vi "Count Change.vi"(1 "reset":bool, 2 "X":variant, 3 "Y":variant) -> (0 "Out":dbl)   [LabVIEW 2019]
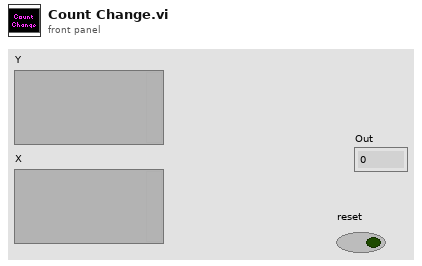
[diagram p1: front panel]
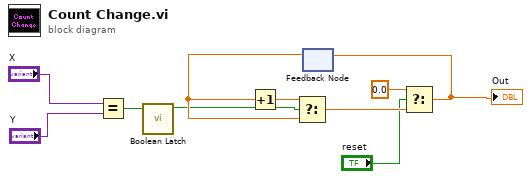
[diagram p0: block diagram]
diagram:
  n1 = Equal?(x="X", y="Y") -> (x = y?=w4:bool)
  n2 = call "Boolean Latch.vi"("Input"=w4) -> ("Output"=w3:bool)  [unwired: 10 in]
  n3 = feedback #1() -> (w7:dbl)  [unwired: 1 in]
  n4 = Increment(x=w7) -> (x+1=w8:dbl)
  n5 = Select(t=w8, s=w3, f=w7) -> (s? t:f=w5:dbl)
  n6 = Select(t=0.0, s="reset", f=w5) -> (s? t:f=w1:dbl)
  "Out" <- w1
  n7 = feedback-in #1(w1) -> ()
